vi "Start.vi"(8 "error in (no error)":errorcluster, 11 "Object ref in":T1) -> (0 "error out":errorcluster, 3 "Object ref out":T1)   [LabVIEW 2013, in "SLMControl.lvlib" / "SC-Main.lvclass"]
uses:
  SC-Main.lvclass
  Object-reference.ctl
  SC-Main.lvclass/SC-Main.ctl
  Application-status.ctl
  UI/Control-names.ctl
  Read UI.vi
  Read Status.vi
  UI/Set-control-enable-multiple.vi
  UI/Set-control-boolean.vi
  UI/SC-UI.lvclass
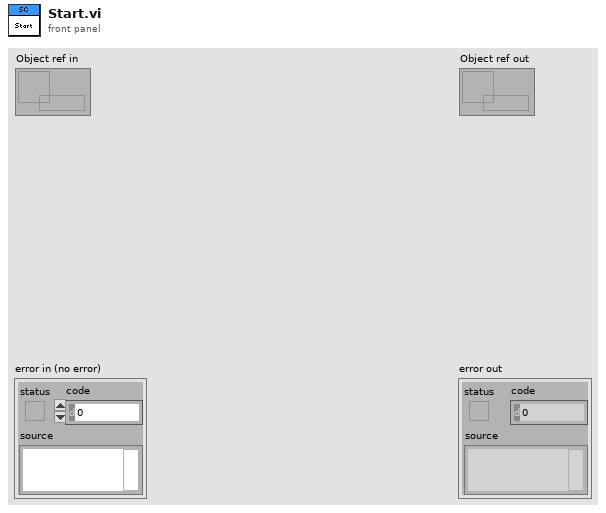
[diagram p1: front panel]
types:
  T1 = typedef "SLMControl.lvlib/SC-Main.lvclass/Object-reference.ctl" = refnum<data-value>
  T2 = typedef "SLMControl.lvlib/SC-UI.lvclass/Control-names.ctl" = enum16{"Com-in", "Com-out", "Help", "Status", "Load configuration", "Save configuration", "Load lasing files", "Load deposition files", "Clear", "Files", "Activate", "Execute", "Abort", "Options", "Current layer", "Current iteration", "Last elapsed time", "Deposition status", "Lasing job", "Status LEDs", "Exiting led", "Initialized led", "Files loaded led", "Activated led", "Executing led", "Deposition led", "Lasing job led", "Lasing led"}
  T3 = typedef "SLMControl.lvlib/SC-Main.lvclass/Application-status.ctl" = enum16{"Idle", "Initialized", "Configured", "Activated", "Started", "Paused", "Stopped", "Reset", "Error", "Exited"}
  T4 = typedef "SLMControl.lvlib/SC-Main.lvclass/Client-status.ctl" = enum16{"Idle", "Initialized", "Configured", "Activated", "Started", "Paused", "Stopped", "Reset", "Error", "Exited"}
  T5 = typedef "SLMControl.lvlib/SC-UI.lvclass/Panes-reference.ctl" = refnum<data-value>
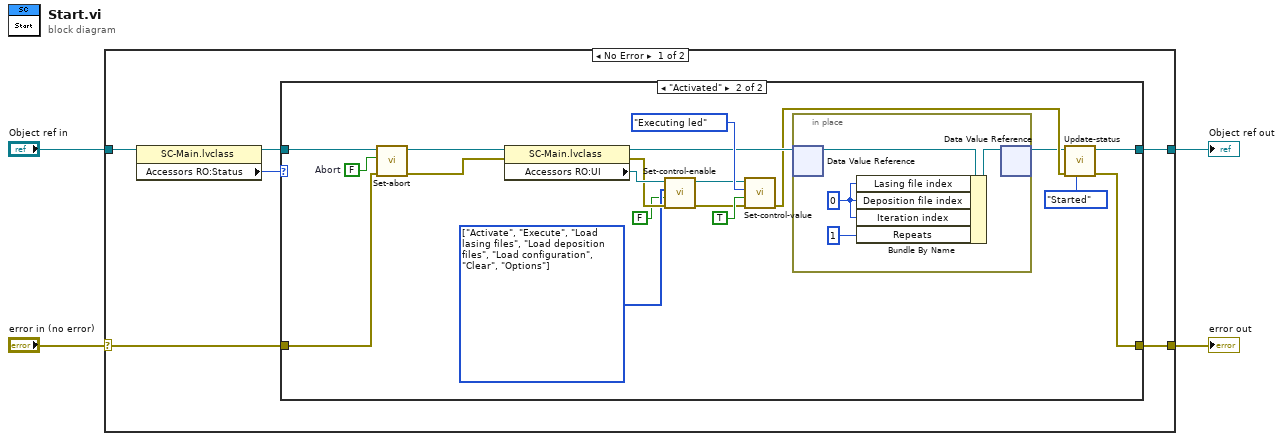
[diagram p0: block diagram]
diagram:
  n1 = case shown="No Error" "error in (no error)" {
    selector: "error in (no error)" -> [w10 w37]
    tunnel: [w9 w37] -> w3
    tunnel: [w8 w36] -> w1
    tunnel: "Object ref in" -> [w7 w36]
    frame No Error {
      n2 = property class="SC-Main.lvclass"(reference=w7) -> (reference out=w6:T1, "Accessors RO:Status"=w5:T4)  [unwired: 1 in, 1 out]
      n3 = case shown="\"Activated\"" w5 {
        tunnel: w6 -> [w12 w30]
        tunnel: w10 -> [w11 w29]
        tunnel: [w11 w27] -> w9
        tunnel: [w12 w26] -> w8
        frame Default {
        }
        frame "Activated" {
          w21 = T2[] [enum."Activate", enum."Execute", enum."Load lasing files", enum."Load deposition files", enum."Load configuration", enum."Clear", enum."Options"] items=["Com-in", "Com-out", "Help", "Status", "Load configuration", "Save configuration", "Load lasing files", "Load deposition files", "Clear", "Files", "Activate", "Execute", "Abort", "Options", "Current layer", "Current iteration", "Last elapsed time", "Deposition status", "Lasing job", "Status LEDs", "Exiting led", "Initialized led", "Files loaded led", "Activated led", "Executing led", "Deposition led", "Lasing job led", "Lasing led"] ("Control names")
          w31 = FALSE  # Abort
          n4 = call "Set-abort.vi"("error in (no error)"=w29, "Abort"=w31, "Object ref in"=w30) -> ("error out"=w13:errorcluster, "Object ref out"=w14:T1)  [unwired: 7 in]
          n5 = property class="SC-Main.lvclass"(reference=w14, error in=w13) -> (reference out=w17:T1, error out=w22:errorcluster, "Accessors RO:UI"=w23:T5)
          n6 = call-poly "Set-control-enable.vi"("error in (no error)"=w22, "Enable?"=FALSE, "Control names"=w21, "Panes in"=w23) -> ("error out"=w18:errorcluster, "Panes out"=w19:T5)  [unwired: 6 in]
          n7 = call-poly "Set-control-value.vi"("error in (no error)"=w18, "Value"=TRUE, "Control name"=Control-names."Executing led", "Panes in"=w19) -> ("error out"=w16:errorcluster)  [unwired: 6 in, 1 out]
          n8 = in-place {
            w33 = 0
            n9 = in-place-dvr #1(w17) -> (w35:refnum<class "SC-Main.lvclass">)  [unwired: 1 out]
            n10 = Bundle By Name(cluster=w35, "Lasing file index"=w33, "Deposition file index"=w33, "Iteration index"=w33, "Repeats"=1 ("Repeats W")) -> (w34:refnum<class "SC-Main.lvclass">)
            n11 = in-place-dvr #1(w34) -> (w15:T1)  [unwired: 1 out]
          }
          n12 = call "Update-status.vi"("Status"=Application-status."Started", "error in (no error)"=w16, "Object ref in"=w15) -> ("error out"=w27:errorcluster, "Object ref out"=w26:T1)  [unwired: 7 in]
        }
      }
    }
    frame Error {
    }
  }
  "error out" <- w3
  "Object ref out" <- w1
